vi "DeleteTag.vi"(0 "reference":refnum<vi>, 1 "Tag":string, 5 "error in (no error)":errorcluster) -> (19 "error out":errorcluster)   [LabVIEW 2017]
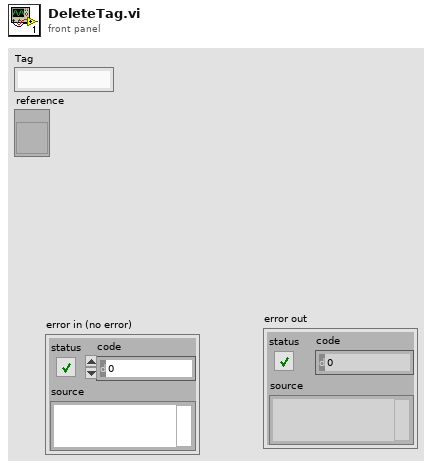
[diagram p1: front panel]
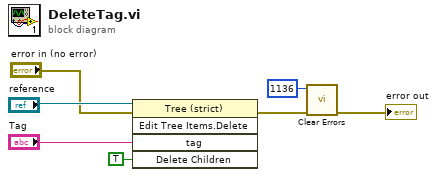
[diagram p0: block diagram]
diagram:
  n1 = invoke class="Tree (strict)" method="Edit Tree Items.Delete"(reference="reference", error in="error in (no error)", "tag"="Tag", "Delete Children"=TRUE ("Delete Children?")) -> (error out=w3:errorcluster)  [unwired: 1 in, 4 out]
  n2 = call <vilib>:"Clear Errors.vi"("error in (no error)"=w3, "specific error code to clear (0: all)"=1136) -> ("error out"=→"error out":errorcluster)  [unwired: 4 in, 1 out]
